vi "Relay.vi"() -> ()   [LabVIEW 2025]
doc: "This example shows how to control a relay.\n\nThis example expects a USB cable connected from your development PC to the Type B USB Jack (next to the power input) on the roboRIO.\n\nThis example requires the Driver Station to be running with Teleoperated Enabled."
uses:
  <vilib>/Rock Robotics/SystemInterfaces/DIO/FPGA_DIORelayChannel.ctl
  <vilib>/Rock Robotics/WPI/Relay/WPI_RelayValue.ctl
  <vilib>/Rock Robotics/WPI/Relay/WPI_RelayDirection.ctl
panel:
  out "SPIKE LED color":u32(colorbox)=1985280
  in  "RelayDirection":T1
  in  "stop":bool
  in  "RelayValue":T2
  in  "RelayChannel":T3
  # "Set these inputs before running."
  # "This can be set while running."
  # "This example requires the Driver Station to be running with Teleoperated Enabled."
  # "Off = Amber\nOn = ---\nForward = Green\nReverse = Red"
  # "Connect\nPower\nHere"
  # "GND"
  # "M-"
  # "Connect\nLoad\nHere"
  # "SPIKE"
  # "12V"
  # "M+"
  # "B"
  # "20A"
  # "PWM cable"
  # "fuse"
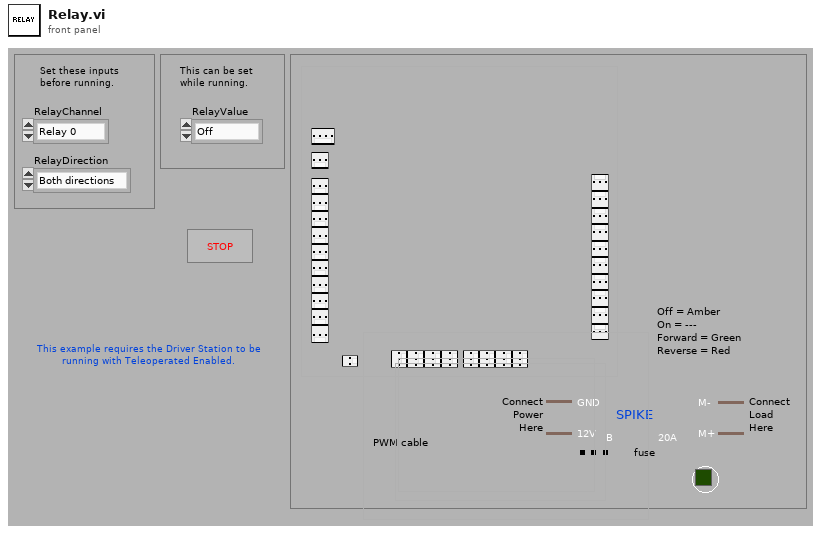
[diagram p1: front panel]
types:
  T1 = typedef "WPI_RelayDirection.ctl" = enum16{"Both directions", "Forward only", "Reverse only"}
  T2 = typedef "WPI_RelayValue.ctl" = enum16{"Off", "On", "Forward", "Reverse"}
  T3 = typedef "FPGA_DIORelayChannel.ctl" = enum8{"Relay 0", "Relay 1", "Relay 2", "Relay 3", "Invalid"}
  T4 = typedef "WPI_RelayDevRef.ctl" = cluster{"DevStatus":errorcluster, "Relay Channel":T3, "Relay Direction":T1}
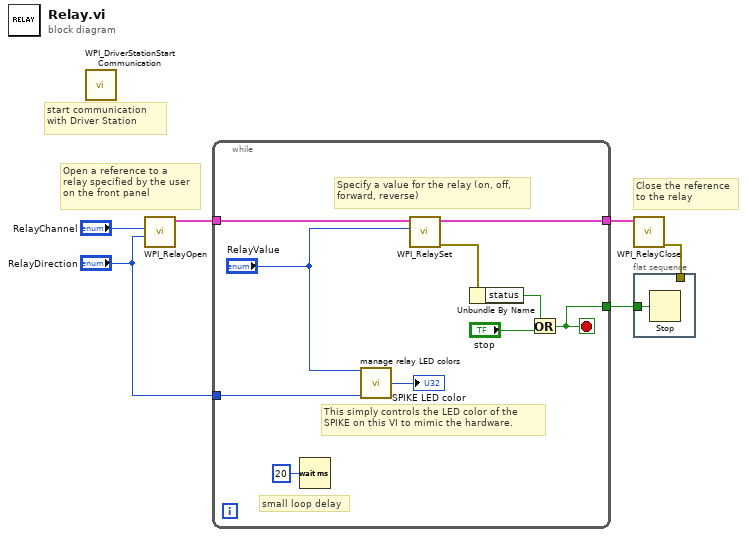
[diagram p0: block diagram]
diagram:
  # "start communication with Driver Station"
  # "Close the reference\nto the relay"
  # "Open a reference to a \nrelay specified by the user\non the front panel"
  n1 = call <vilib>:"WPI_DriverStationStart Communication.vi"() -> ()  [unwired: 3 in, 9 out]
  n2 = call <vilib>:"WPI_RelayOpen.vi"("Relay Direction"="RelayDirection", "Relay Channel"="RelayChannel") -> ("RelayDevRef"=w6:T4)  [unwired: 1 in, 8 out]
  n3 = while {
    tunnel: w6 -> [w16]
    tunnel: [w15] -> w5
    tunnel: [w10] -> w2
    tunnel: "RelayDirection" -> [w8]
    stop <- w10 stop-if-true
    # "This simply controls the LED color of the SPIKE on this VI to mimic the hardware."
    # "small loop delay"
    # "Specify a value for the relay (on, off, \nforward, reverse)"
    n4 = Wait (ms)(milliseconds to wait=u32 20) -> ()  [unwired: 1 out]
    n5 = call "manage relay LED colors.vi"("RelayValue"="RelayValue", "RelayDirection"=w8) -> ("LED color"=→"SPIKE LED color":u32)  [unwired: 13 in]
    n6 = call <vilib>:"WPI_RelaySet.vi"("RelayValue"="RelayValue", "RelayDevRef"=w16) -> ("error out"=w13:errorcluster, "RelayDevRef"=w15:T4)  [unwired: 1 in, 7 out]
    n7 = Unbundle By Name(w13) -> ("status"=w11:bool)
    n8 = Or(x=w11, y="stop") -> (x .or. y?=w10:bool)
  }
  n9 = call <vilib>:"WPI_RelayClose.vi"("RelayDevRef"=w5) -> ("error out"=w1:errorcluster)  [unwired: 1 in, 9 out]
  n10 = flat-sequence {
    tunnel: w2 -> [w17]
    tunnel: w1 -> [_]
    frame #0 {
      n11 = Stop(stop? (T)=w17) -> ()
    }
  }
